vi "03.1 Event-driven User Interface.vi"() -> ()   [LabVIEW 2019]
panel:
  out "Current Time 2":timestamp format="%<%x %.3X>T"
  in  "Check Time 2":bool
  out "Temperature (ºF) 2":dbl
  in  "Temperature (ºC) 2":dbl
  in  "Stop 2":bool
  in  "Acquire":bool
  out "Graph":dbl[][](graph)
  out "Data":dbl[][](graph)
  in  "Stop":bool
  out "Current Time":timestamp format="%<%x %.3X>T"
  in  "Acquire Data":bool
  in  "Check Time":bool
  out "Temperature (ºF)":dbl
  in  "Temperature (ºC)":dbl
  # "POLLING"
  # "EVENT-DRIVEN"
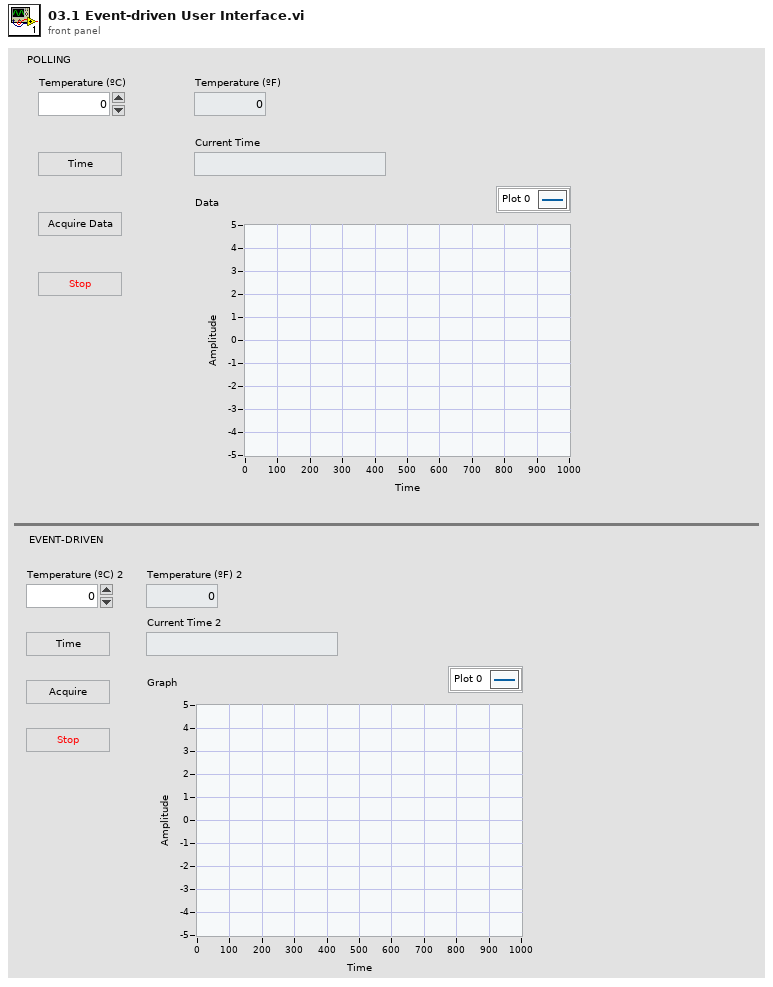
[diagram p1: front panel]
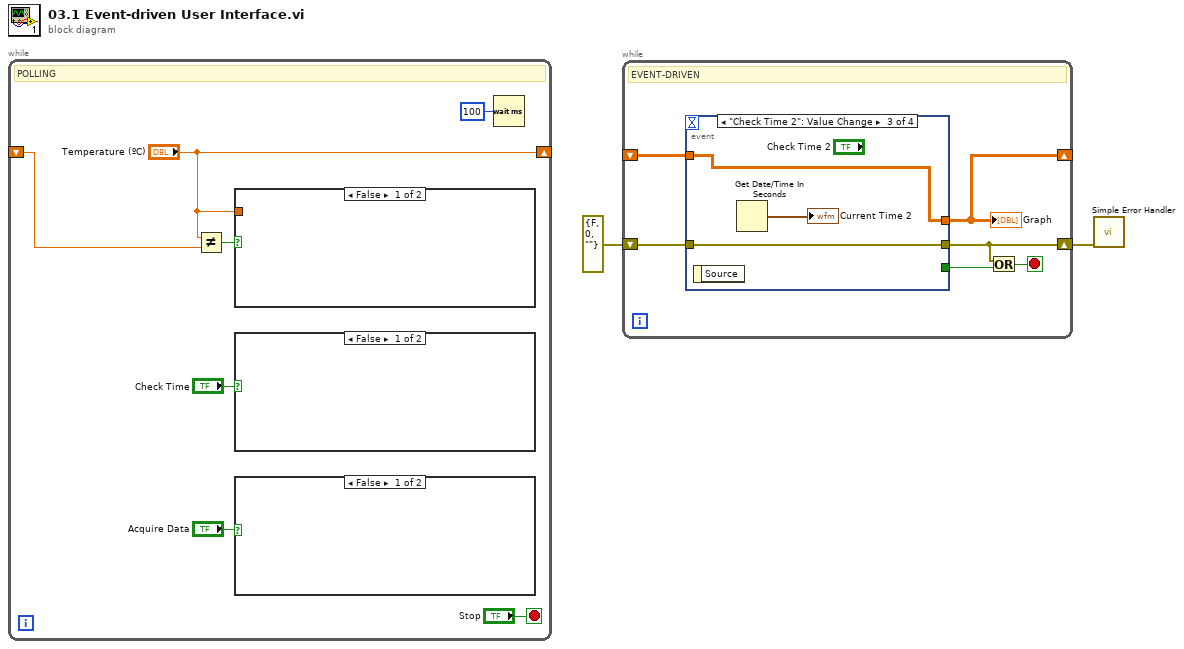
[diagram p0: block diagram]
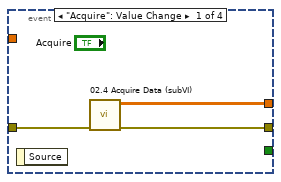
[diagram p2: hidden frame]
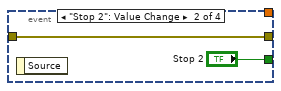
[diagram p3: hidden frame]
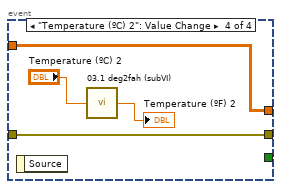
[diagram p4: hidden frame]
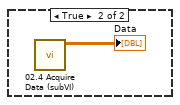
[diagram p5: hidden frame]
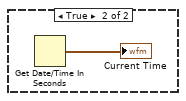
[diagram p6: hidden frame]
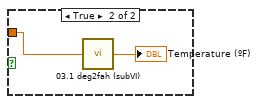
[diagram p7: hidden frame]
diagram:
  n1 = while {
    shift-right: ["Temperature (ºC)"] -> _
    shift-left: _ -> [w7]
    stop <- "Stop" stop-if-true
    # "POLLING"
    n2 = Not Equal?(x="Temperature (ºC)", y=w7) -> (x != y?=w8:bool)
    n3 = case shown="False" w8 {
      tunnel: "Temperature (ºC)" -> [_ w13]
      frame False {
      }
      frame True {
        n4 = call "03.1 deg2fah (subVI).vi"("Degrees"=w13) -> ("Fahrenheit"=→"Temperature (ºF)":dbl)
      }
    }
    n5 = case shown="False" "Check Time" {
      frame False {
      }
      frame True {
        n6 = Get Date/Time In Seconds() -> (seconds since 1Jan1904=→"Current Time":timestamp)
      }
    }
    n7 = case shown="False" "Acquire Data" {
      frame False {
      }
      frame True {
        n8 = call "02.4 Acquire Data (subVI).vi"() -> ("2D DBL"=→"Data":dbl[][])  [unwired: 10 in, 1 out]
      }
    }
    n9 = Wait (ms)(milliseconds to wait=u32 100) -> ()  [unwired: 1 out]
  }
  n10 = while {
    shift-right: [w17] -> w2
    shift-left: errorcluster {"status"=FALSE, "code"=0, "source"=""} ("error constant") -> [w19]
    shift-right: [w16] -> _
    shift-left: _ -> [w15]
    stop <- w18 stop-if-true
    # "EVENT-DRIVEN"
    n11 = event shown="[2] \"Check Time 2\": Value Change" {
      selector: _ -> [_ _ _ _]
      dyn-events: _ -> [_ _ _ _]
      timeout: _ -> [_ _ _ _]
      tunnel: w19 -> [w21 w24 w26 w29]
      tunnel: [w20 w24 w26 w29] -> w17
      tunnel: [w22 _ w25 w28] -> w16
      tunnel: w15 -> [_ _ w25 w28]
      tunnel: [_ "Stop 2" _ _] -> w14
      event "Acquire": Value Change {
        n12 = event-data() -> ()  [unwired: 1 in, 1 out]
        n13 = call "02.4 Acquire Data (subVI).vi"("Error In"=w21) -> ("error out"=w20:errorcluster, "2D DBL"=w22:dbl[][])  [unwired: 9 in]
      }
      event "Stop 2": Value Change {
        n14 = event-data() -> ()  [unwired: 1 in, 1 out]
      }
      event "Check Time 2": Value Change {
        n15 = event-data() -> ()  [unwired: 1 in, 1 out]
        n16 = Get Date/Time In Seconds() -> (seconds since 1Jan1904=→"Current Time 2":timestamp)
      }
      event "Temperature (ºC) 2": Value Change {
        n17 = event-data() -> ()  [unwired: 1 in, 1 out]
        n18 = call "03.1 deg2fah (subVI).vi"("Degrees"="Temperature (ºC) 2") -> ("Fahrenheit"=→"Temperature (ºF) 2":dbl)
      }
    }
    "Graph" <- w16
    n19 = Or(x=w17, y=w14) -> (x .or. y?=w18:bool)
  }
  n20 = call <vilib>:"Simple Error Handler.vi"("error in (no error)"=w2) -> ()  [unwired: 4 in, 5 out]
